vi "AccelnetTorqueOutScale.vi"(1 "Demand torque (Nm)":dbl) -> (0 "Torque setpoint to drive":i16)   [LabVIEW 2018]
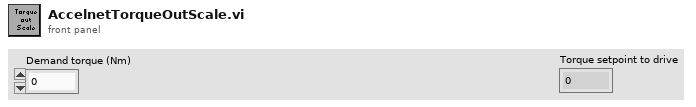
[diagram p1: front panel]
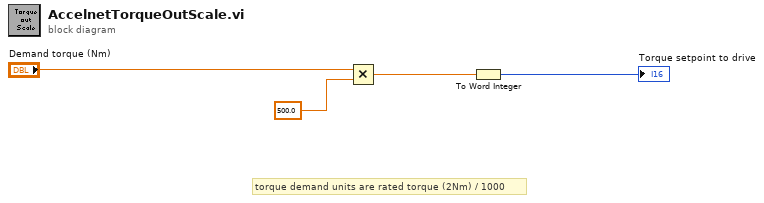
[diagram p0: block diagram]
diagram:
  # "torque demand units are rated torque (2Nm) / 1000"
  n1 = Multiply(x="Demand torque (Nm)", y=500.0) -> (x*y=w1:dbl)
  n2 = To Word Integer(number=w1) -> (16bit integer=→"Torque setpoint to drive":i16)
